vi "SerialNumber to DeviceName_modified.vi"(8 "error in (no error)":errorcluster, 9 "NI2 Serial Number":i64 format="%x", 10 "NI1 Serial Number":i64 format="%x") -> (0 "error out":errorcluster, 1 "NI2 Device Name":tag, 2 "NI1 Device Name":tag)   [LabVIEW 2017]
uses:
  <resource>/objmgr/daqmx.rc
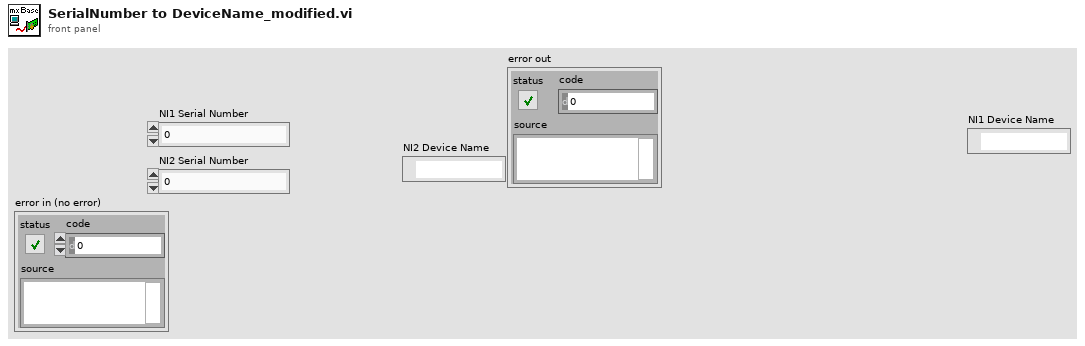
[diagram p1: front panel]
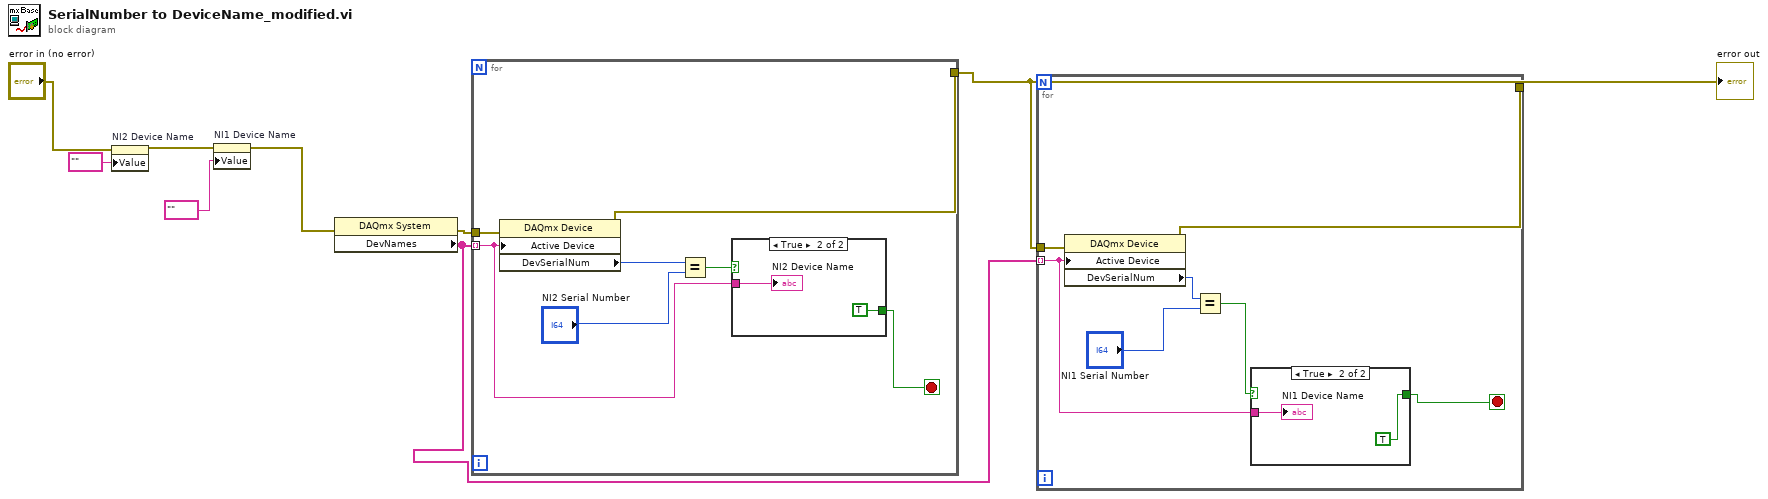
[diagram p0: block diagram]
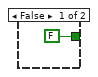
[diagram p2: hidden frame]
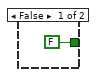
[diagram p3: hidden frame]
diagram:
  n1 = property on="NI2 Device Name" class="DAQmxName"(error in="error in (no error)", "Value"=tag "" ("NI2 Device Name")) -> (error out=w5:errorcluster)  [unwired: 1 in, 1 out]
  n2 = property on="NI1 Device Name" class="DAQmxName"(error in=w5, "Value"=tag "" ("NI1 Device Name 2")) -> (error out=w4:errorcluster)  [unwired: 1 in, 1 out]
  n3 = property class="DAQmx System"(error in=w4) -> (error out=w8:errorcluster, "DevNames"=w6:tag[])  [unwired: 1 in, 1 out]
  n4 = for {
    tunnel: w6 -> [w12] mode=indexing
    tunnel: w8 -> [w15]
    tunnel: [w14] -> w7
    stop <- w10 stop-if-true
    n5 = property class="DAQmx Device"(error in=w15, "Active Device"=w12) -> (error out=w14:errorcluster, "DevSerialNum"=w13:u32)  [unwired: 1 in, 1 out]
    n6 = Equal?(x=w13, y="NI2 Serial Number") -> (x = y?=w11:bool)
    n7 = case shown="True" w11 {
      tunnel: w12 -> [_ w18]
      tunnel: [FALSE TRUE] -> w10
      frame False {
      }
      frame True {
        "NI2 Device Name" <- w18
      }
    }
  }
  "error out" <- w7
  n8 = for {
    tunnel: w6 -> [w22] mode=indexing
    tunnel: w7 -> [w25]
    tunnel: [w24] -> _
    stop <- w20 stop-if-true
    n9 = property class="DAQmx Device"(error in=w25, "Active Device"=w22) -> (error out=w24:errorcluster, "DevSerialNum"=w23:u32)  [unwired: 1 in, 1 out]
    n10 = Equal?(x=w23, y="NI1 Serial Number") -> (x = y?=w21:bool)
    n11 = case shown="True" w21 {
      tunnel: w22 -> [_ w28]
      tunnel: [FALSE TRUE] -> w20
      frame False {
      }
      frame True {
        "NI1 Device Name" <- w28
      }
    }
  }
